vi "Scripting_FindTypeDefsOnDiagram.vi"(0 "ViRef":refnum<vi>, 1 "TypeDefConstantsToSearchSearchFor":path[](array[path]), 5 "error in (no error)":errorcluster) -> (15 "BlockDiagramConstantsFound":refnum<vi>[](array[refnum]), 19 "error out":errorcluster)   [LabVIEW 2014]
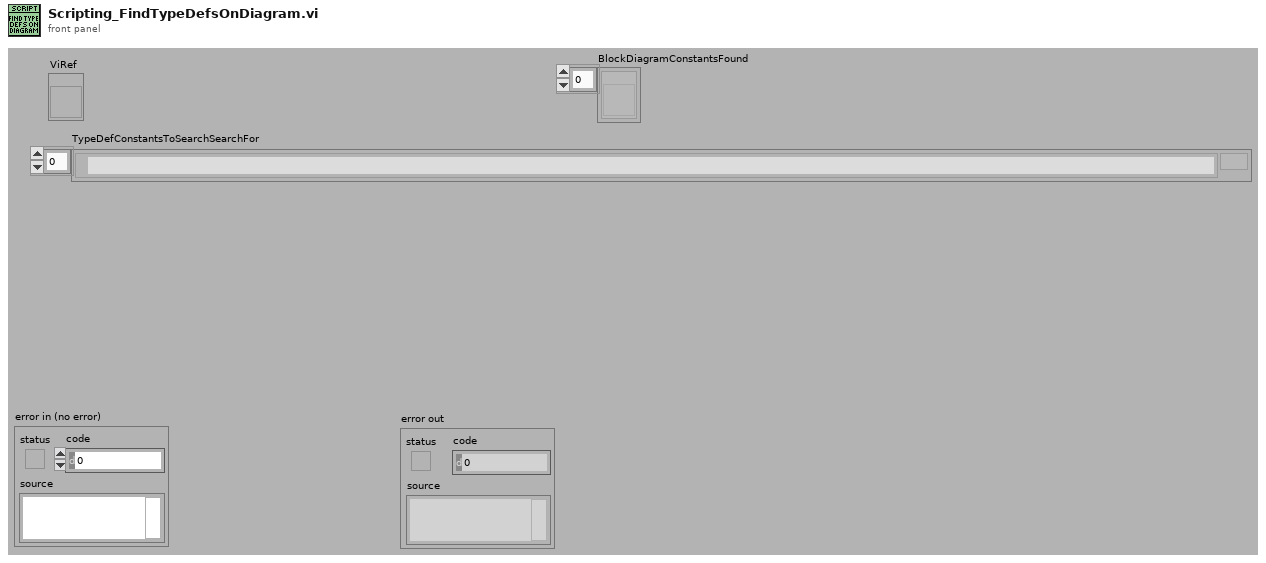
[diagram p1: front panel]
types:
  T1 = enum32{"not a typedef", "typedef", "strict typedef", "class private data"}
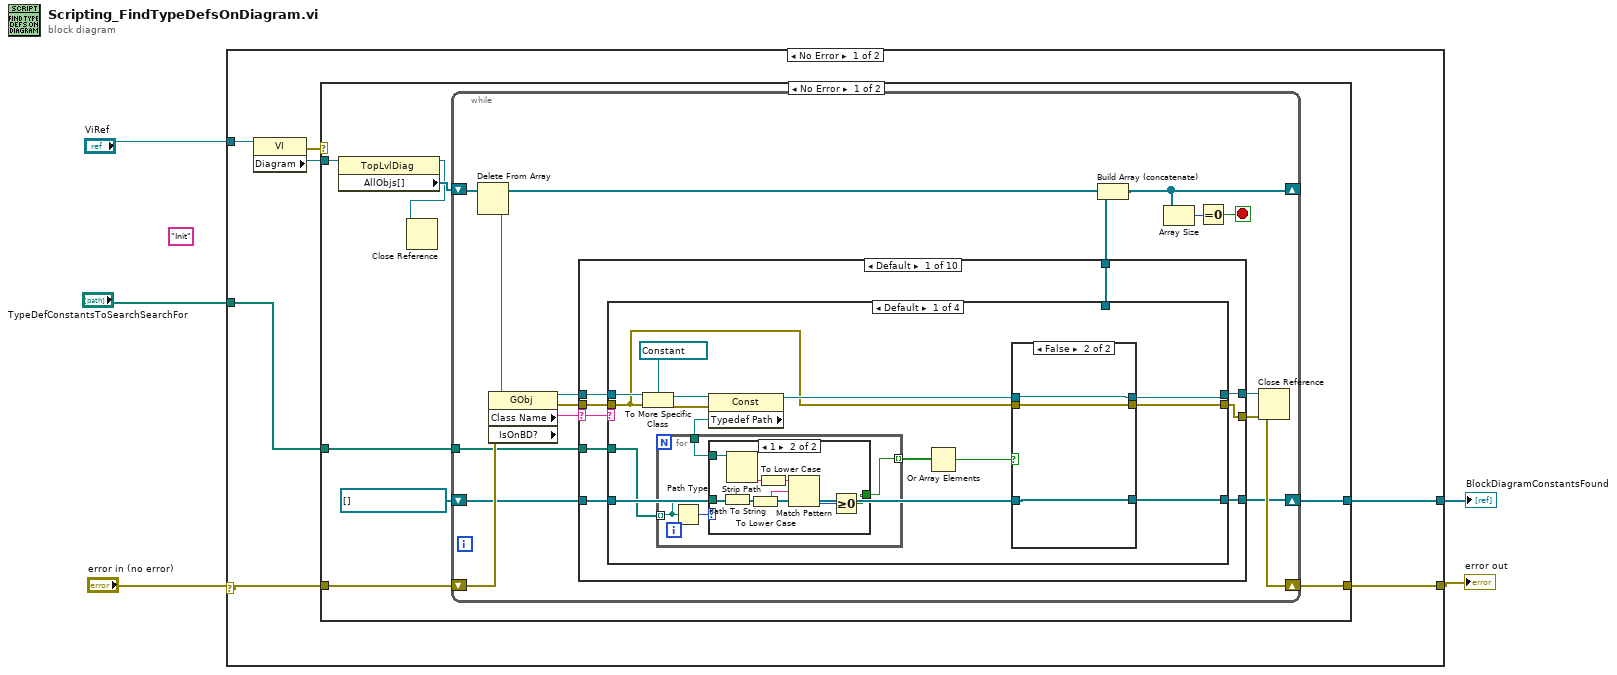
[diagram p0: block diagram]
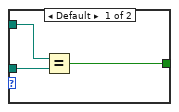
[diagram p2: hidden frame]
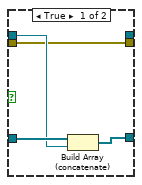
[diagram p3: hidden frame]
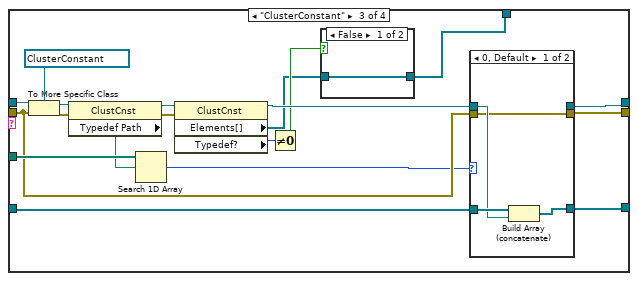
[diagram p5: hidden frame]
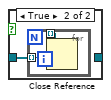
[diagram p6: hidden frame]
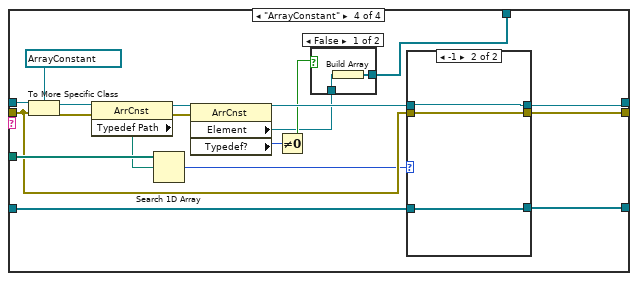
[diagram p8: hidden frame]
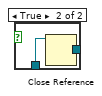
[diagram p9: hidden frame]
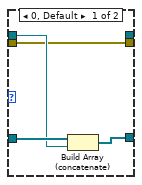
[diagram p10: hidden frame]
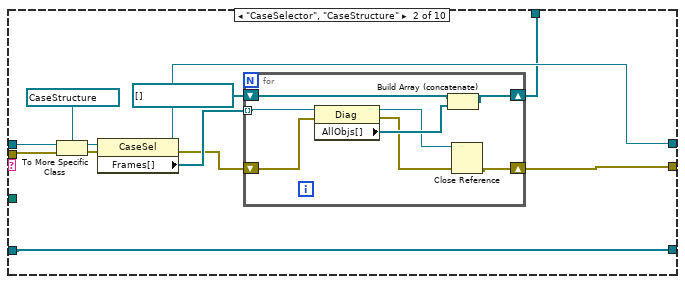
[diagram p11: hidden frame]
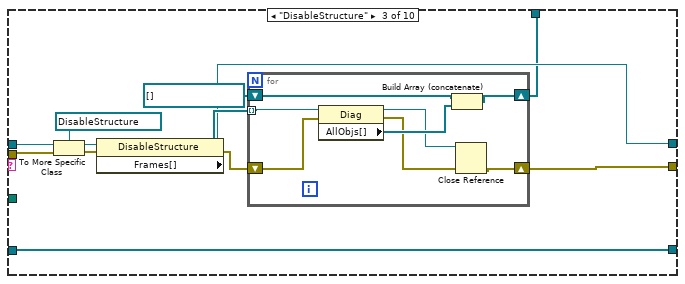
[diagram p12: hidden frame]
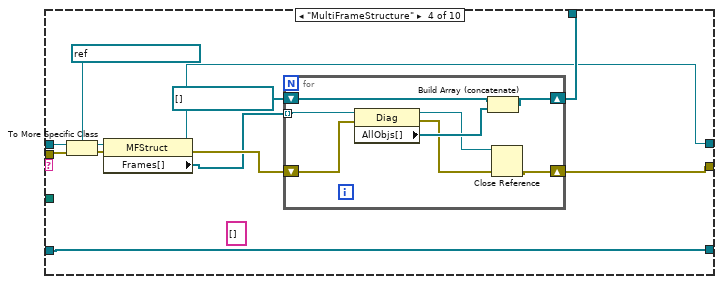
[diagram p13: hidden frame]
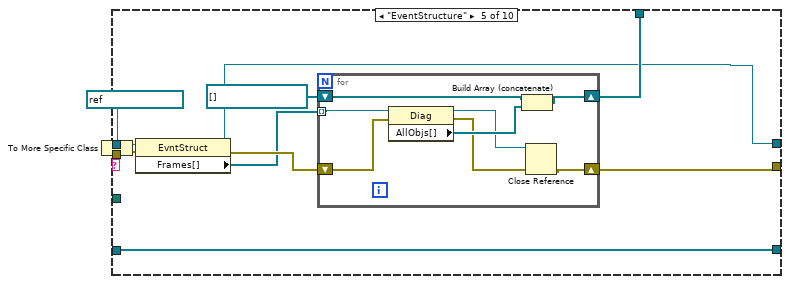
[diagram p14: hidden frame]
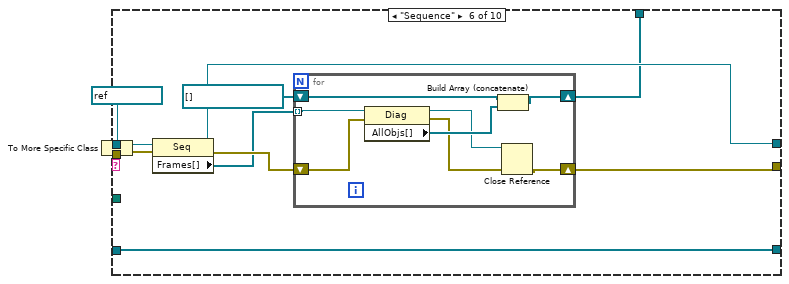
[diagram p15: hidden frame]
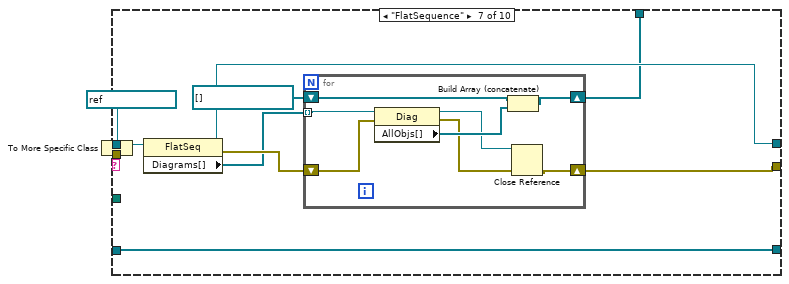
[diagram p16: hidden frame]
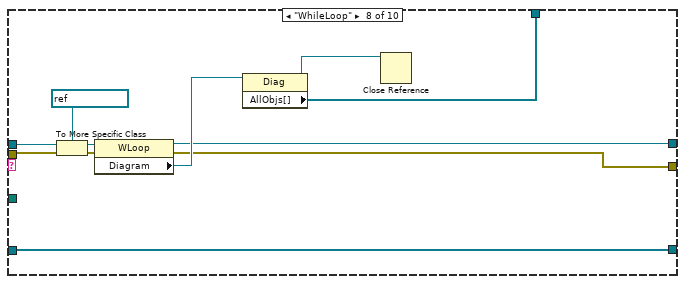
[diagram p17: hidden frame]
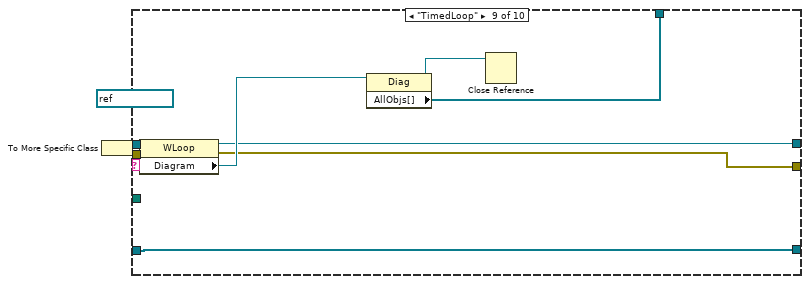
[diagram p18: hidden frame]
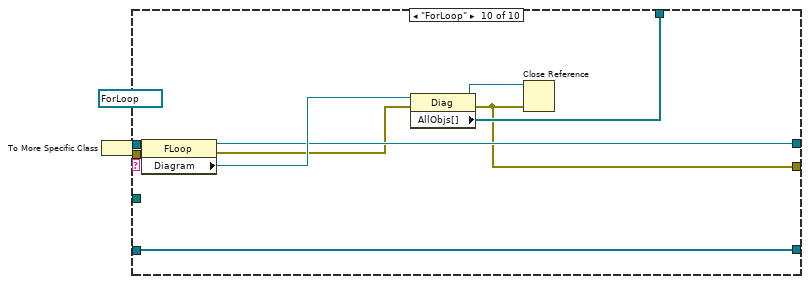
[diagram p19: hidden frame]
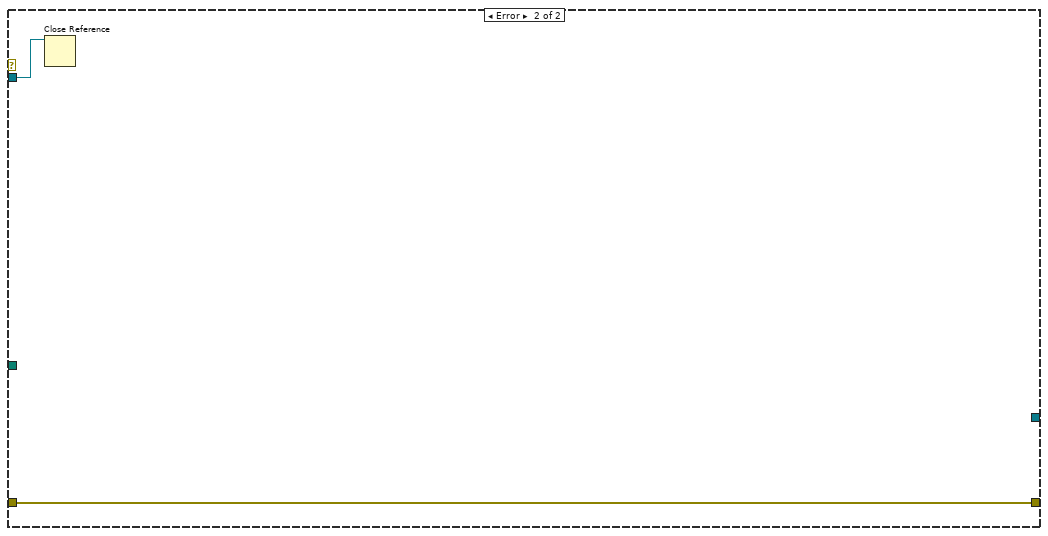
[diagram p20: hidden frame]
diagram:
  (unwired) "Init"
  n1 = case shown="No Error" "error in (no error)" {
    selector: "error in (no error)" -> [w7 w298]
    tunnel: [w12 w298] -> w5
    tunnel: "TypeDefConstantsToSearchSearchFor" -> [w11 _]
    tunnel: "ViRef" -> [w10 _]
    tunnel: [w6 _] -> w1
    frame No Error {
      n2 = property class="VI"(reference=w10) -> (error out=w8:errorcluster, "Diagram"=w9:refnum<vi>)  [unwired: 1 in, 1 out]
      n3 = case shown="No Error" w8 {
        tunnel: w9 -> [w20 w296]
        tunnel: [w18 w297] -> w12
        tunnel: w7 -> [w17 w297]
        tunnel: w11 -> [w16 _]
        tunnel: [w13 _] -> w6
        frame No Error {
          n4 = property class="TopLvlDiag"(reference=w20) -> (reference out=w15:refnum<vi>, "AllObjs[]"=w19:refnum<vi>[])  [unwired: 1 in, 1 out]
          n5 = Close Reference(reference=w15) -> ()  [unwired: 1 in, 1 out]
          n6 = while {
            shift-right: [w28] -> _
            shift-left: w19 -> [w36]
            shift-right: [w23] -> w18
            shift-left: w17 -> [w25]
            tunnel: w16 -> [w24]
            shift-right: [w21] -> w13
            shift-left: refnum<vi>[] [] -> [w22]
            stop <- w34 stop-if-true
            n7 = Delete From Array(array=w36) -> (deleted portion=w30:refnum<vi>, array with subset deleted=w29:refnum<vi>[])  [unwired: 2 in]
            n8 = property class="GObj" props=["Class Name", "IsOnBD?"](reference=w30, error in=w25) -> (reference out=w32:refnum<vi>, error out=w33:errorcluster, "Class Name"=w31:string)  [unwired: 1 out]
            n9 = case shown="Default" w31 {
              selector: w31 -> [w45 _ _ _ _ _ _ _ _ _]
              tunnel: w32 -> [w43 w154 w174 w194 w214 w234 w253 w272 w283 w295]
              tunnel: w33 -> [w44 w149 w169 w191 w211 w231 w252 w268 w279 w291]
              tunnel: [w40 w147 w167 w184 w205 w227 w245 w264 w275 w286] -> w23
              tunnel: [w37 w145 w165 w186 w206 w225 w244 w266 w277 w289] -> w27
              tunnel: [w41 w148 w168 w185 w204 w226 w246 w265 w276 w288] -> w26
              tunnel: w24 -> [w42 _ _ _ _ _ _ _ _ _]
              tunnel: w22 -> [w39 w143 w163 w183 w203 w223 w243 w262 w273 w284]
              tunnel: [w38 w143 w163 w183 w203 w223 w243 w262 w273 w284] -> w21
              frame Default {
                n10 = case shown="Default" w45 {
                  tunnel: w44 -> [w46 w84 w96 w125]
                  tunnel: w43 -> [w59 w83 w103 w132]
                  tunnel: [w58 w84 w97 w126] -> w40
                  tunnel: [w57 w83 w92 w118] -> w41
                  tunnel: w42 -> [w50 _ w99 w128]
                  tunnel: w39 -> [w52 w82 w95 w120]
                  tunnel: [w51 w82 w93 w117] -> w38
                  tunnel: [_ _ w86 w114] -> w37
                  frame Default {
                    n11 = To More Specific Class(target class=refnum<vi> refnum ("WhileLoop"), reference=w59, error in=w46) -> (specific class reference=w55:refnum<vi>, error out=w54:errorcluster)
                    n12 = property class="Const"(reference=w55, error in=w54) -> (reference out=w53:refnum<vi>, "Typedef Path"=w49:path)  [unwired: 1 out]
                    n13 = for {
                      tunnel: w50 -> [w62] mode=indexing
                      tunnel: w49 -> [w61]
                      tunnel: [w60] -> w48 mode=indexing
                      n14 = Path Type(1:w62) -> (0:w63:i16)
                      n15 = case shown="1" w63 {
                        tunnel: w62 -> [w66 w74]
                        tunnel: w61 -> [w65 w73]
                        tunnel: [w64 w69] -> w60
                        frame Default {
                          n16 = Equal?(x=w65, y=w66) -> (x = y?=w64:bool)
                        }
                        frame 1 {
                          n17 = Path To String(path=w74) -> (string=w71:string)
                          n18 = Strip Path(path=w73) -> (name=w72:string)  [unwired: 1 out]
                          n19 = To Lower Case(string=w71) -> (all lower case string=w67:string)
                          n20 = To Lower Case(string=w72) -> (all lower case string=w68:string)
                          n21 = Match Pattern(string=w68, regular expression=w67) -> (offset past match=w70:i32)  [unwired: 1 in, 3 out]
                          n22 = Greater Or Equal To 0?(x=w70) -> (x >= 0?=w69:bool)
                        }
                      }
                    }
                    n23 = Or Array Elements(Boolean array=w48) -> (logical OR=w47:bool)
                    n24 = case shown="False" w47 {
                      tunnel: w46 -> [w75 w80]
                      tunnel: w53 -> [w76 w81]
                      tunnel: [_ w81] -> w57
                      tunnel: [w75 w80] -> w58
                      tunnel: w52 -> [w78 w79]
                      tunnel: [w77 w79] -> w51
                      frame True {
                        n25 = Build Array (concatenate)(w78, w76) -> (w77:refnum<vi>[])
                      }
                      frame False {
                      }
                    }
                  }
                  frame "PolymorphicSubVI", "SubVI" {
                  }
                  frame "ClusterConstant" {
                    n26 = To More Specific Class(target class=refnum<vi> refnum ("WhileLoop"), reference=w103, error in=w96) -> (specific class reference=w101:refnum<vi>, error out=w100:errorcluster)
                    n27 = property class="ClustCnst"(reference=w101, error in=w100) -> (reference out=w90:refnum<vi>, error out=w91:errorcluster, "Typedef Path"=w98:path)
                    n28 = Search 1D Array(1D array=w99, element=w98) -> (index of element=w94:i32)  [unwired: 1 in]
                    n29 = property class="ClustCnst"(reference=w90, error in=w91) -> (reference out=w89:refnum<vi>, "Elements[]"=w85:refnum<vi>[], "Typedef?"=w88:T1)  [unwired: 1 out]
                    n30 = Not Equal To 0?(x=w88) -> (x != 0?=w87:bool)
                    n31 = case shown="False" w87 {
                      tunnel: [w104 _] -> w86
                      tunnel: w85 -> [w104 w105]
                      frame False {
                      }
                      frame True {
                        n32 = for {
                          tunnel: [w106] -> _ mode=indexing
                          tunnel: w105 -> [w106] mode=indexing
                          n33 = Close Reference(reference=w106) -> ()  [unwired: 1 in, 1 out]
                        }
                      }
                    }
                    n34 = case shown="0, Default" w94 {
                      tunnel: w96 -> [w107 w112]
                      tunnel: w89 -> [w108 w113]
                      tunnel: [_ w113] -> w92
                      tunnel: [w107 w112] -> w97
                      tunnel: w95 -> [w110 w111]
                      tunnel: [w109 w111] -> w93
                      frame 0, Default {
                        n35 = Build Array (concatenate)(w110, w108) -> (w109:refnum<vi>[])
                      }
                      frame -1 {
                      }
                    }
                  }
                  frame "ArrayConstant" {
                    n36 = To More Specific Class(target class=refnum<vi> refnum ("WhileLoop"), reference=w132, error in=w125) -> (specific class reference=w130:refnum<vi>, error out=w129:errorcluster)
                    n37 = property class="ArrCnst"(reference=w130, error in=w129) -> (reference out=w123:refnum<vi>, error out=w122:errorcluster, "Typedef Path"=w127:path)
                    n38 = Search 1D Array(1D array=w128, element=w127) -> (index of element=w121:i32)  [unwired: 1 in]
                    n39 = property class="ArrCnst"(reference=w123, error in=w122) -> (reference out=w119:refnum<vi>, "Element"=w115:refnum<vi>, "Typedef?"=w124:T1)  [unwired: 1 out]
                    n40 = Not Equal To 0?(x=w124) -> (x != 0?=w116:bool)
                    n41 = case shown="False" w116 {
                      tunnel: w115 -> [w134 w135]
                      tunnel: [w133 _] -> w114
                      frame False {
                        n42 = Build Array(w134) -> (w133:refnum<vi>[])
                      }
                      frame True {
                        n43 = Close Reference(reference=w135) -> ()  [unwired: 1 in, 1 out]
                      }
                    }
                    n44 = case shown="-1" w121 {
                      tunnel: w125 -> [w136 w141]
                      tunnel: w119 -> [w137 w142]
                      tunnel: [_ w142] -> w118
                      tunnel: [w136 w141] -> w126
                      tunnel: w120 -> [w139 w140]
                      tunnel: [w138 w140] -> w117
                      frame 0, Default {
                        n45 = Build Array (concatenate)(w139, w137) -> (w138:refnum<vi>[])
                      }
                      frame -1 {
                      }
                    }
                  }
                }
              }
              frame "CaseSelector", "CaseStructure" {
                n46 = To More Specific Class(target class=refnum<vi> refnum ("CaseSelector"), reference=w154, error in=w149) -> (specific class reference=w152:refnum<vi>, error out=w150:errorcluster)
                n47 = property class="CaseSel"(reference=w152, error in=w150) -> (reference out=w148:refnum<vi>, error out=w146:errorcluster, "Frames[]"=w151:refnum<vi>[])
                n48 = for {
                  tunnel: w151 -> [w162] mode=indexing
                  shift-right: [w155] -> w147
                  shift-left: w146 -> [w161]
                  shift-right: [w158] -> w145
                  shift-left: refnum<vi>[] [] -> [w160]
                  n49 = property class="Diag"(reference=w162, error in=w161) -> (reference out=w156:refnum<vi>, error out=w157:errorcluster, "AllObjs[]"=w159:refnum<vi>[])
                  n50 = Build Array (concatenate)(w160, w159) -> (w158:refnum<vi>[])
                  n51 = Close Reference(reference=w156, error in (no error)=w157) -> (error out=w155:errorcluster)
                }
              }
              frame "DisableStructure" {
                n52 = To More Specific Class(target class=refnum<vi> refnum ("CaseSelector"), reference=w174, error in=w169) -> (specific class reference=w172:refnum<vi>, error out=w170:errorcluster)
                n53 = property class="DisableStructure"(reference=w172, error in=w170) -> (reference out=w168:refnum<vi>, error out=w166:errorcluster, "Frames[]"=w171:refnum<vi>[])
                n54 = for {
                  tunnel: w171 -> [w182] mode=indexing
                  shift-right: [w175] -> w167
                  shift-left: w166 -> [w181]
                  shift-right: [w178] -> w165
                  shift-left: refnum<vi>[] [] -> [w180]
                  n55 = property class="Diag"(reference=w182, error in=w181) -> (reference out=w176:refnum<vi>, error out=w177:errorcluster, "AllObjs[]"=w179:refnum<vi>[])
                  n56 = Build Array (concatenate)(w180, w179) -> (w178:refnum<vi>[])
                  n57 = Close Reference(reference=w176, error in (no error)=w177) -> (error out=w175:errorcluster)
                }
              }
              frame "MultiFrameStructure" {
                (unwired) string[] []
                n58 = To More Specific Class(target class=refnum<vi> refnum ("MultiFrameStructure"), reference=w194, error in=w191) -> (specific class reference=w193:refnum<vi>, error out=w192:errorcluster)
                n59 = property class="MFStruct"(reference=w193, error in=w192) -> (reference out=w185:refnum<vi>, error out=w188:errorcluster, "Frames[]"=w187:refnum<vi>[])
                n60 = for {
                  tunnel: w187 -> [w202] mode=indexing
                  shift-right: [w195] -> w184
                  shift-left: w188 -> [w201]
                  shift-right: [w198] -> w186
                  shift-left: refnum<vi>[] [] -> [w200]
                  n61 = property class="Diag"(reference=w202, error in=w201) -> (reference out=w196:refnum<vi>, error out=w197:errorcluster, "AllObjs[]"=w199:refnum<vi>[])
                  n62 = Build Array (concatenate)(w200, w199) -> (w198:refnum<vi>[])
                  n63 = Close Reference(reference=w196, error in (no error)=w197) -> (error out=w195:errorcluster)
                }
              }
              frame "EventStructure" {
                n64 = To More Specific Class(target class=refnum<vi> refnum ("EventStructure"), reference=w214, error in=w211) -> (specific class reference=w213:refnum<vi>, error out=w212:errorcluster)
                n65 = property class="EvntStruct"(reference=w213, error in=w212) -> (reference out=w204:refnum<vi>, error out=w208:errorcluster, "Frames[]"=w207:refnum<vi>[])
                n66 = for {
                  tunnel: w207 -> [w222] mode=indexing
                  shift-right: [w215] -> w205
                  shift-left: w208 -> [w221]
                  shift-right: [w218] -> w206
                  shift-left: refnum<vi>[] [] -> [w220]
                  n67 = property class="Diag"(reference=w222, error in=w221) -> (reference out=w216:refnum<vi>, error out=w217:errorcluster, "AllObjs[]"=w219:refnum<vi>[])
                  n68 = Build Array (concatenate)(w220, w219) -> (w218:refnum<vi>[])
                  n69 = Close Reference(reference=w216, error in (no error)=w217) -> (error out=w215:errorcluster)
                }
              }
              frame "Sequence" {
                n70 = To More Specific Class(target class=refnum<vi> refnum ("Sequence"), reference=w234, error in=w231) -> (specific class reference=w233:refnum<vi>, error out=w232:errorcluster)
                n71 = property class="Seq"(reference=w233, error in=w232) -> (reference out=w226:refnum<vi>, error out=w228:errorcluster, "Frames[]"=w224:refnum<vi>[])
                n72 = for {
                  tunnel: w224 -> [w242] mode=indexing
                  shift-right: [w235] -> w227
                  shift-left: w228 -> [w241]
                  shift-right: [w238] -> w225
                  shift-left: refnum<vi>[] [] -> [w240]
                  n73 = property class="Diag"(reference=w242, error in=w241) -> (reference out=w236:refnum<vi>, error out=w237:errorcluster, "AllObjs[]"=w239:refnum<vi>[])
                  n74 = Build Array (concatenate)(w240, w239) -> (w238:refnum<vi>[])
                  n75 = Close Reference(reference=w236, error in (no error)=w237) -> (error out=w235:errorcluster)
                }
              }
              frame "FlatSequence" {
                n76 = To More Specific Class(target class=refnum<vi> refnum ("FlatSequence"), reference=w253, error in=w252) -> (specific class reference=w250:refnum<vi>)  [unwired: 1 out]
                n77 = property class="FlatSeq"(reference=w250) -> (reference out=w246:refnum<vi>, error out=w248:errorcluster, "Diagrams[]"=w247:refnum<vi>[])  [unwired: 1 in]
                n78 = for {
                  tunnel: w247 -> [w261] mode=indexing
                  shift-right: [w254] -> w245
                  shift-left: w248 -> [w260]
                  shift-right: [w257] -> w244
                  shift-left: refnum<vi>[] [] -> [w259]
                  n79 = property class="Diag"(reference=w261, error in=w260) -> (reference out=w255:refnum<vi>, error out=w256:errorcluster, "AllObjs[]"=w258:refnum<vi>[])
                  n80 = Build Array (concatenate)(w259, w258) -> (w257:refnum<vi>[])
                  n81 = Close Reference(reference=w255, error in (no error)=w256) -> (error out=w254:errorcluster)
                }
              }
              frame "WhileLoop" {
                n82 = To More Specific Class(target class=refnum<vi> refnum ("WhileLoop"), reference=w272, error in=w268) -> (specific class reference=w271:refnum<vi>, error out=w269:errorcluster)
                n83 = property class="WLoop"(reference=w271, error in=w269) -> (reference out=w265:refnum<vi>, error out=w264:errorcluster, "Diagram"=w267:refnum<vi>)
                n84 = property class="Diag"(reference=w267) -> (reference out=w263:refnum<vi>, "AllObjs[]"=w266:refnum<vi>[])  [unwired: 1 in, 1 out]
                n85 = Close Reference(reference=w263) -> ()  [unwired: 1 in, 1 out]
              }
              frame "TimedLoop" {
                n86 = To More Specific Class(target class=refnum<vi> refnum ("WhileLoop"), reference=w283, error in=w279) -> (specific class reference=w282:refnum<vi>, error out=w280:errorcluster)
                n87 = property class="WLoop"(reference=w282, error in=w280) -> (reference out=w276:refnum<vi>, error out=w275:errorcluster, "Diagram"=w278:refnum<vi>)
                n88 = property class="Diag"(reference=w278) -> (reference out=w274:refnum<vi>, "AllObjs[]"=w277:refnum<vi>[])  [unwired: 1 in, 1 out]
                n89 = Close Reference(reference=w274) -> ()  [unwired: 1 in, 1 out]
              }
              frame "ForLoop" {
                n90 = To More Specific Class(target class=refnum<vi> refnum ("WhileLoop"), reference=w295, error in=w291) -> (specific class reference=w294:refnum<vi>, error out=w292:errorcluster)
                n91 = property class="FLoop"(reference=w294, error in=w292) -> (reference out=w288:refnum<vi>, error out=w287:errorcluster, "Diagram"=w290:refnum<vi>)
                n92 = property class="Diag"(reference=w290, error in=w287) -> (reference out=w285:refnum<vi>, error out=w286:errorcluster, "AllObjs[]"=w289:refnum<vi>[])
                n93 = Close Reference(reference=w285, error in (no error)=w286) -> ()  [unwired: 1 out]
              }
            }
            n94 = Build Array (concatenate)(w29, w27) -> (w28:refnum<vi>[])
            n95 = Array Size(array=w28) -> (size(s)=w35:i32)
            n96 = Equal To 0?(x=w35) -> (x = 0?=w34:bool)
            n97 = Close Reference(reference=w26, error in (no error)=w23) -> ()  [unwired: 1 out]
          }
        }
        frame Error {
          n98 = Close Reference(reference=w296) -> ()  [unwired: 1 in, 1 out]
        }
      }
    }
    frame Error {
    }
  }
  "error out" <- w5
  "BlockDiagramConstantsFound" <- w1
